vi "All hand commands.vi"() -> ()   [LabVIEW 2016]
panel:
  out "Finger 5 (little)":dbl(knob) scale=0.0..180.0
  out "Finger 3 (middle)":dbl(knob) scale=0.0..180.0
  out "Finger 4 (ring)":dbl(knob) scale=0.0..180.0
  out "Finger 2 (index)":dbl(knob) scale=0.0..180.0
  out "Finger 1 (thumb)":dbl(knob) scale=0.0..180.0
  out "Finger 5 (individual)":bool
  out "Finger 4 (individual)":bool
  out "Finger 3 (individual)":bool
  out "Finger 2 (individual)":bool
  out "Finger 1 (individual)":bool
  in  "Finger 5 (individual)":bool
  in  "FInger 4 (individual)":bool
  in  "Finger 3 (individual)":bool
  in  "Finger 2 (individual)":bool
  in  "Finger 1 (individual)":bool
  in  "stop":bool
  out "Test 4":bool
  out "Test 3":bool
  out "Test 2":bool
  out "Test 1":bool
  in  "Boolean 2":bool
  in  "Boolean 1":bool
  # "comp3\nNeurotechnology"
  # "Booleans representing the first two\nbits in message from comp2"
  # "Gauge (mätare) displaying\neach finger angle"
  # "Booleans for the last five bits\ncontrolling individual fingers"
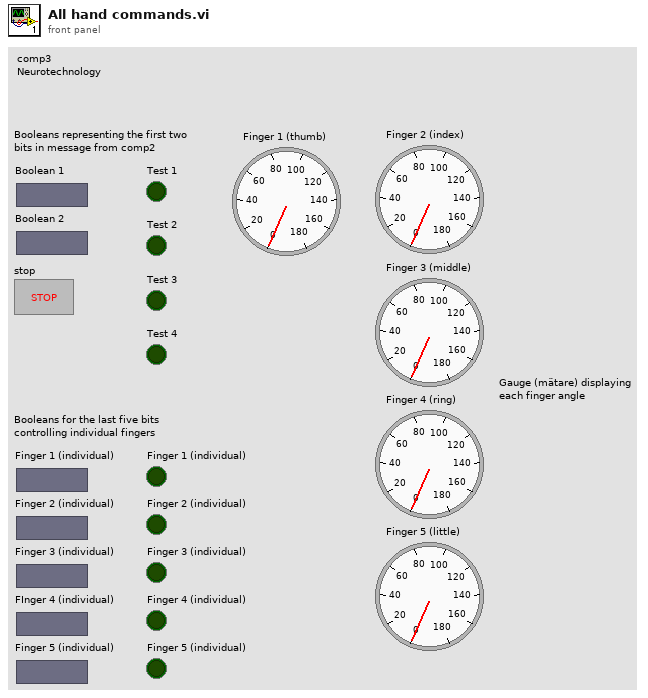
[diagram p1: front panel]
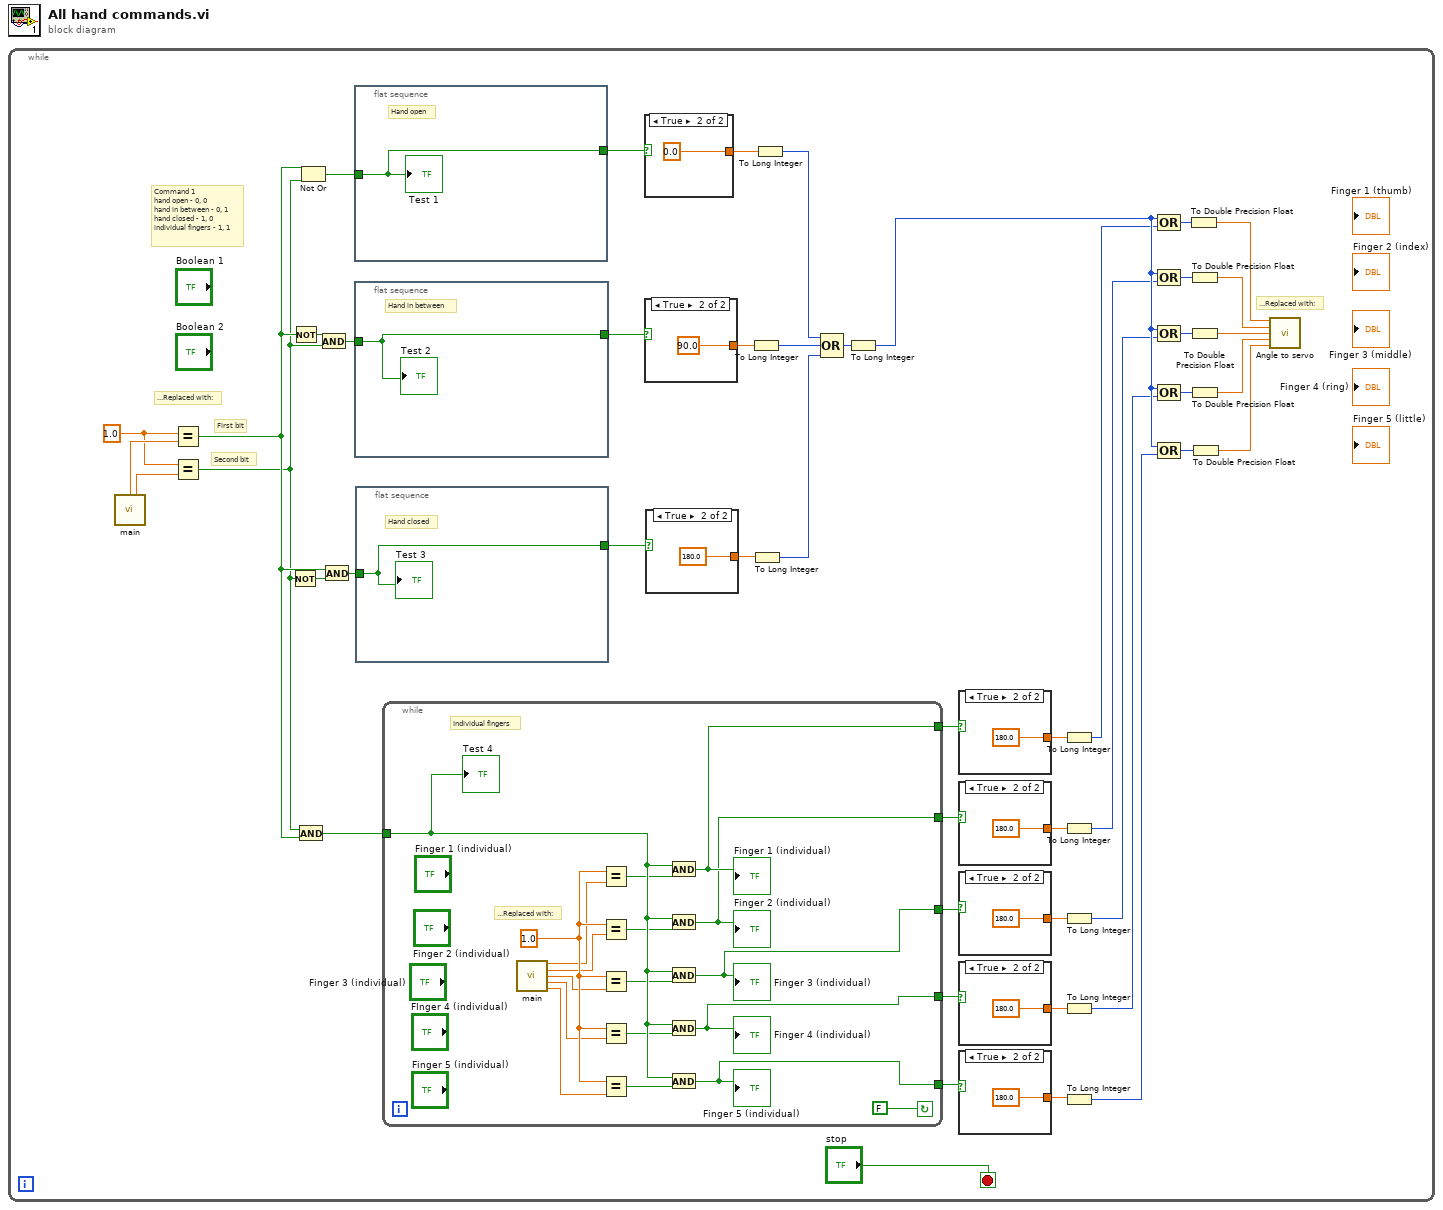
[diagram p0: block diagram]
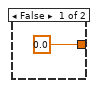
[diagram p2: hidden frame]
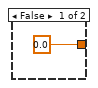
[diagram p3: hidden frame]
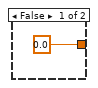
[diagram p4: hidden frame]
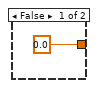
[diagram p5: hidden frame]
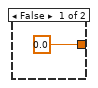
[diagram p6: hidden frame]
diagram:
  n1 = while {
    stop <- "stop" stop-if-true
    w17 = 1.0
    # "...Replaced with:"
    # "...Replaced with:"
    # "Second bit"
    # "First bit"
    # "Command 1\nhand open - 0, 0\nhand in between - 0, 1\nhand closed - 1, 0\nindividual fingers - 1, 1"
    n2 = call "main.vi"() -> ("Bit1"=w20:dbl, "Bit2"=w18:dbl)  [unwired: 9 in, 5 out]
    n3 = Equal?(x=w17, y=w20) -> (x = y?=w19:bool)
    n4 = Equal?(x=w17, y=w18) -> (x = y?=w16:bool)
    n5 = Not(x=w16) -> (.not. x?=w47:bool)
    n6 = Not(x=w19) -> (.not. x?=w48:bool)
    n7 = And(x=w16, y=w19) -> (x .and. y?=w46:bool)
    n8 = Not Or(1:w16, 2:w19) -> (0:w45:bool)
    n9 = And(x=w48, y=w16) -> (x .and. y?=w44:bool)
    n10 = And(x=w19, y=w47) -> (x .and. y?=w42:bool)
    n11 = flat-sequence {
      tunnel: w45 -> [w64]
      tunnel: [w64] -> w39
      frame #0 {
        # "Hand open"
        "Test 1" <- w64
      }
    }
    n12 = flat-sequence {
      tunnel: w44 -> [w63]
      tunnel: [w63] -> w41
      frame #0 {
        # "Hand in between"
        "Test 2" <- w63
      }
    }
    n13 = flat-sequence {
      tunnel: w42 -> [w62]
      tunnel: [w62] -> w37
      frame #0 {
        # "Hand closed"
        "Test 3" <- w62
      }
    }
    n14 = while {
      tunnel: w46 -> [w82]
      tunnel: [w80] -> w15
      tunnel: [w79] -> w14
      tunnel: [w78] -> w13
      tunnel: [w77] -> w12
      tunnel: [w76] -> w11
      stop <- FALSE continue-if-true
      w75 = 1.0
      # "...Replaced with:"
      # "Individual fingers"
      n15 = call "main.vi"() -> ("BitLittle"=w74:dbl, "BitRing"=w73:dbl, "BitMiddle"=w72:dbl, "BitPointy"=w71:dbl, "BitThumb"=w70:dbl)  [unwired: 9 in, 2 out]
      n16 = Equal?(x=w75, y=w74) -> (x = y?=w69:bool)
      n17 = Equal?(x=w75, y=w73) -> (x = y?=w68:bool)
      n18 = Equal?(x=w75, y=w72) -> (x = y?=w67:bool)
      n19 = Equal?(x=w75, y=w71) -> (x = y?=w66:bool)
      n20 = Equal?(x=w75, y=w70) -> (x = y?=w65:bool)
      n21 = And(x=w82, y=w69) -> (x .and. y?=w80:bool)
      "Finger 1 (individual)" <- w80
      n22 = And(x=w82, y=w68) -> (x .and. y?=w79:bool)
      "Finger 2 (individual)" <- w79
      n23 = And(x=w82, y=w67) -> (x .and. y?=w78:bool)
      "Finger 3 (individual)" <- w78
      n24 = And(x=w82, y=w66) -> (x .and. y?=w77:bool)
      "Finger 4 (individual)" <- w77
      n25 = And(x=w82, y=w65) -> (x .and. y?=w76:bool)
      "Finger 5 (individual)" <- w76
      "Test 4" <- w82
    }
    n26 = case shown="True" w39 {
      tunnel: [_ 0.0] -> w38
      frame False {
      }
      frame True {
      }
    }
    n27 = case shown="True" w41 {
      tunnel: [_ 90.0] -> w40
      frame False {
      }
      frame True {
      }
    }
    n28 = case shown="True" w37 {
      tunnel: [_ 180.0] -> w34
      frame False {
      }
      frame True {
      }
    }
    n29 = To Long Integer(number=w40) -> (32bit integer=w35:i32)
    n30 = To Long Integer(number=w34) -> (32bit integer=w33:i32)
    n31 = To Long Integer(number=w38) -> (32bit integer=w36:i32)
    n32 = Compound Arithmetic op=OR(w36, w35, w33) -> (w32:i32)
    n33 = To Long Integer(number=w32) -> (32bit integer=w31:i32)
    n34 = case shown="True" w15 {
      tunnel: [0.0 180.0] -> w6
      frame False {
      }
      frame True {
      }
    }
    n35 = case shown="True" w14 {
      tunnel: [0.0 180.0] -> w7
      frame False {
      }
      frame True {
      }
    }
    n36 = case shown="True" w13 {
      tunnel: [0.0 180.0] -> w8
      frame False {
      }
      frame True {
      }
    }
    n37 = case shown="True" w12 {
      tunnel: [0.0 180.0] -> w9
      frame False {
      }
      frame True {
      }
    }
    n38 = case shown="True" w11 {
      tunnel: [0.0 180.0] -> w10
      frame False {
      }
      frame True {
      }
    }
    n39 = To Long Integer(number=w6) -> (32bit integer=w25:i32)
    n40 = To Long Integer(number=w7) -> (32bit integer=w24:i32)
    n41 = To Long Integer(number=w8) -> (32bit integer=w23:i32)
    n42 = To Long Integer(number=w9) -> (32bit integer=w22:i32)
    n43 = To Long Integer(number=w10) -> (32bit integer=w21:i32)
    n44 = Compound Arithmetic op=OR(w31, w25) -> (w30:i32)
    n45 = Compound Arithmetic op=OR(w31, w24) -> (w29:i32)
    n46 = Compound Arithmetic op=OR(w31, w23) -> (w28:i32)
    n47 = Compound Arithmetic op=OR(w31, w22) -> (w27:i32)
    n48 = Compound Arithmetic op=OR(w31, w21) -> (w26:i32)
    n49 = To Double Precision Float(number=w30) -> (double precision float=w5:dbl)
    n50 = To Double Precision Float(number=w29) -> (double precision float=w4:dbl)
    n51 = To Double Precision Float(number=w28) -> (double precision float=w3:dbl)
    n52 = To Double Precision Float(number=w27) -> (double precision float=w2:dbl)
    n53 = To Double Precision Float(number=w26) -> (double precision float=w1:dbl)
    n54 = call "Angle to servo.vi"("Angle in degrees finger 1"=w5, "Angle in degrees finger 2"=w4, "Angle in degrees finger 3"=w3, "Angle in degrees finger 4"=w2, "Angle in degrees finger 5"=w1) -> ()  [unwired: 11 in]
  }
